vi "Collect fast fpga metadata.vi"(0 "reference in":refnum<class "metadata.lvclass">, 5 "error in (no error)":errorcluster) -> (14 "reference out":refnum<class "metadata.lvclass">, 16 "Metadata":T1, 17 "Property Names":string[](array[string]), 18 "Property values":string[](array[string]), 19 "error out":errorcluster)   [LabVIEW 2019, in "metadata.lvclass"]
uses:
  metadata.lvclass
  Metadata output --cluster.ctl
  Write time and date string --constant.ctl
panel:
  out "List property names":string
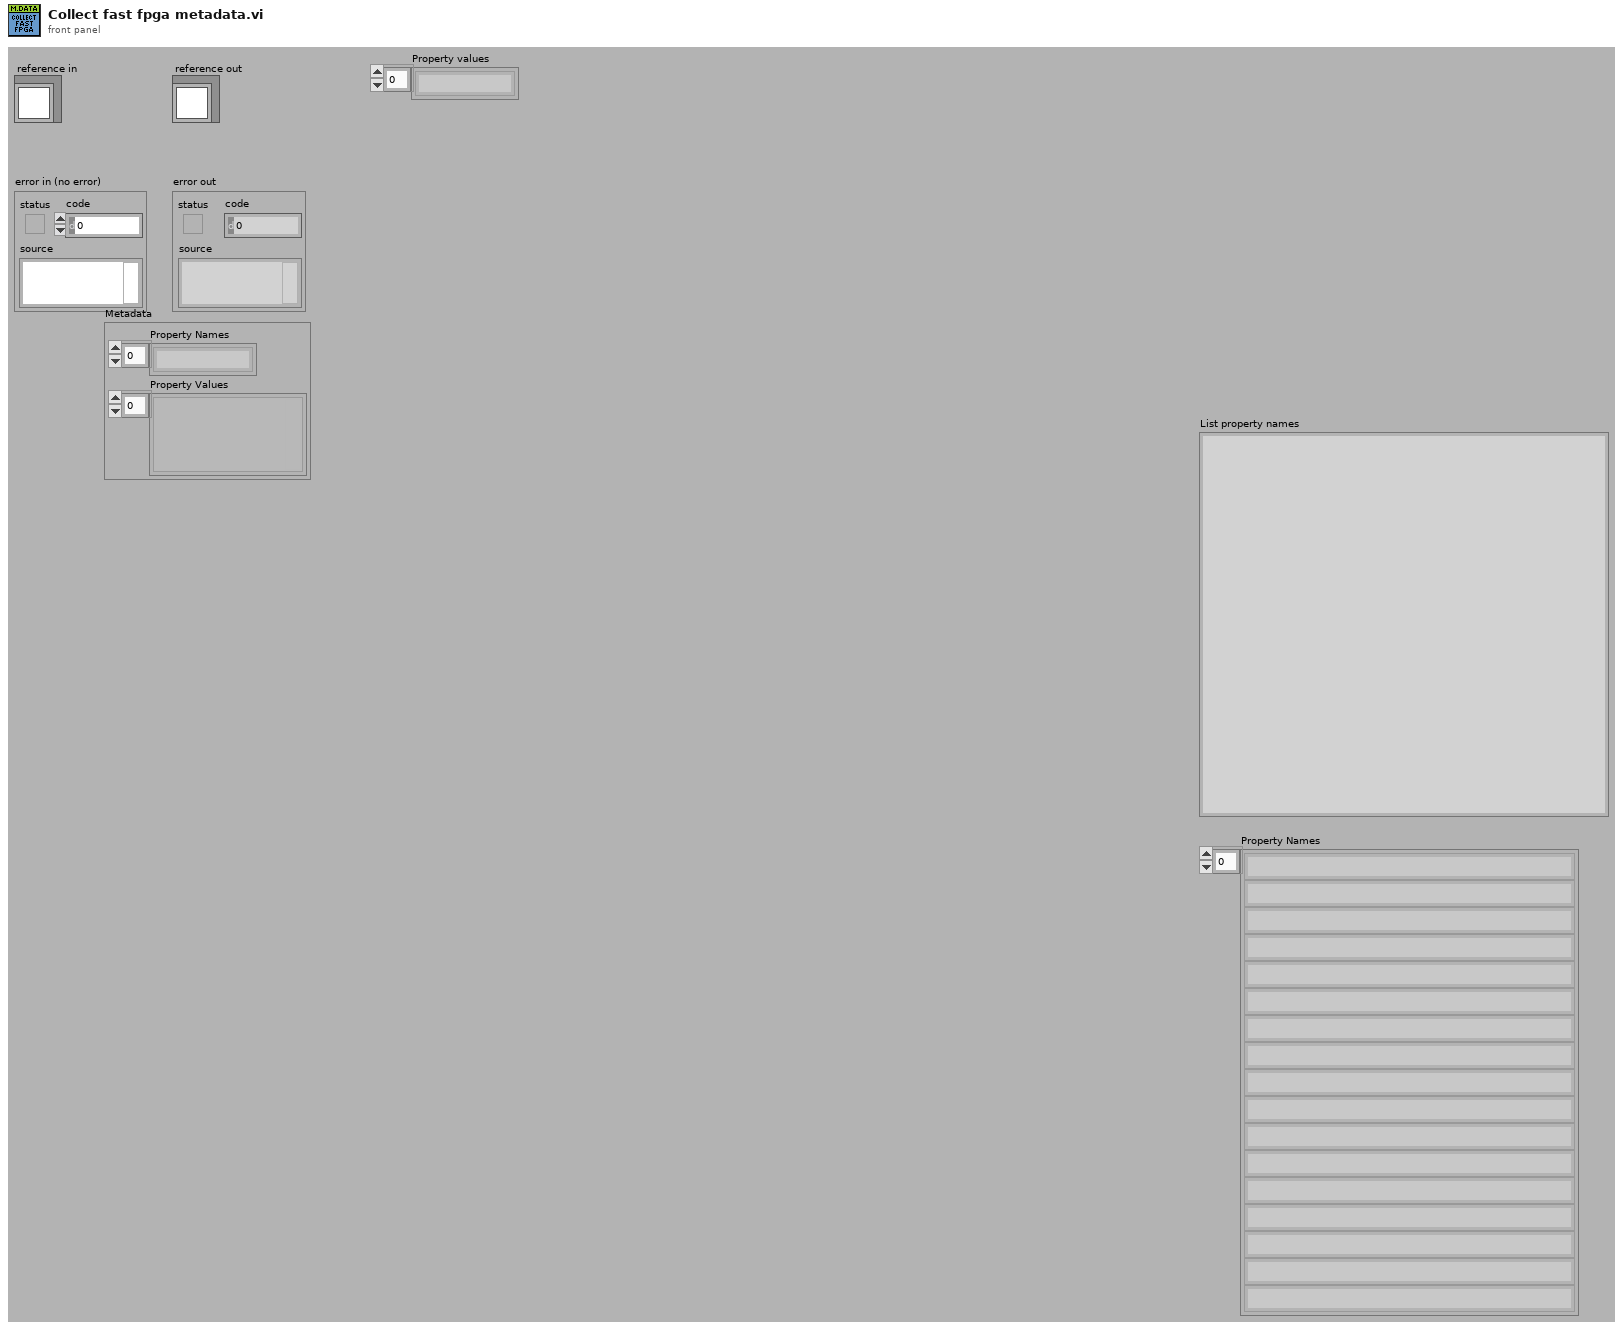
[diagram p1: front panel]
types:
  T1 = typedef "metadata.lvclass/Metadata output --cluster.ctl" = cluster{"Property Names":string[], "Property Values":variant[]}
  T2 = typedef "metadata.lvclass/Write time and date string --constant.ctl" = string
  T3 = typedef "metadata.lvclass/ObjectAttributes.ctl" = cluster{"MyAttribute":dbl, "System Control":T4, "file info":T5, "Sample info":T6, "Cantilever info":T7, "XYZ piezos":T8, "Mapping":T9, "Fcurve segment":T10[], "Fast fpga segment":T12, "Chirp":T13, "precision (6)":i16, "width (-)":i16, "Metadata":T1, "config filepath":path, "Section names []":string[], "Property names []":string[], "nb elements":u16}
  T4 = typedef "metadata.lvclass/System control parameters.ctl" = cluster{"FPGA SW version":string, "TDMS file version":string, "Instrument":string, "Instrument model":string, "Instrument scanner":string, "Instrument clockrate (Mhz)":string, "Instrument tick time (us)":string}
  T5 = typedef "metadata.lvclass/File info parameters.ctl" = cluster{"Time Stamp":timestamp, "Filename":string, "Filepath":path, "User":string, "Experiment_name":string, "Curve_id":string, "number_segments":u8, "number_consecutive_scans":u32}
  T6 = typedef "metadata.lvclass/Sample info parameters.ctl" = cluster{"Sample name":string, "Sample species":string}
  T7 = typedef "metadata.lvclass/Cantilever info parameters.ctl" = cluster{"spring constant calib method":string, "invOLS calib method":string, "thermal calib deflection channel":string, "model":string, "shape":string, "tip geometry":string, "Laser sum (V)":dbl, "Laser power (mA)":dbl, "invOLS_(nm/V)":dbl, "spring constant nominal (N/m)":dbl, "spring constant calib (N/m)":dbl, "resosnance frequency air calib (Hz)":dbl, "resosnance frequency calib (Hz)":dbl, "quality factor":dbl, "Acoefficident_GCI_(nN.s^1.3/m)":dbl, "half angle (deg)":dbl, "tip radius (m)":dbl, "tip height (m)":dbl, "system mount angle (deg)":dbl}
  T8 = typedef "metadata.lvclass/XYZ piezos parameters.ctl" = cluster{"X stage piezo sensitivity (nm/V)":dbl, "X stage piezo gain":dbl, "X velocity (V/tick)":dbl, "X closed loop":bool, "Y stage piezo sensitivity (nm/V)":dbl, "Y stage piezo gain":dbl, "Y velocity (V/tick)":dbl, "Y closed loop":bool, "Z stage piezo sensitivity (nm/V)":dbl, "Z stage piezo gain":dbl, "Z closed loop":bool, "X position (V)":dbl, "Y position (V)":dbl}
  T9 = typedef "metadata.lvclass/Mapping parameters.ctl" = cluster{"Mapping":bool, "index":u16, "position row":u16, "position column":u16, "next position row":i16, "next position column":i16, "X initial position (V)":dbl, "Y initial position (V)":dbl, "X step size (V)":dbl, "Y step size (V)":dbl}
  T10 = typedef "metadata.lvclass/Fcurve segment.ctl" = cluster{"type":T11, "fast_fpga_trigger":bool, "nb":u8, "duration (ticks)":i64, "nb points":i32, "sampling rate (S/s)":u32, "Zpiezo control out":string, "initial deflection (V)":dbl, "relative setpoint":bool, "setpoint on":bool, "setpoint (V)":dbl, "setpoint trigger channel":string, "velocity (V/tick)":dbl, "Z position setpoint trigger (V)":dbl, "Z retract length (V)":dbl, "dec factor":u32}
  T11 = typedef "metadata.lvclass/Segment type--combobox.ctl" = string
  T12 = typedef "metadata.lvclass/fast fpga segment parameters.ctl" = cluster{"Fast start time trigger":timestamp, "nb_points":u32, "sampling_rate_(S/s)":u32, "duration_(ticks)":u32}
  T13 = typedef "metadata.lvclass/Chirp added parameters.ctl" = cluster{"f start (Hz)":dbl, "f end (Hz)":dbl, "Sweep type":string}
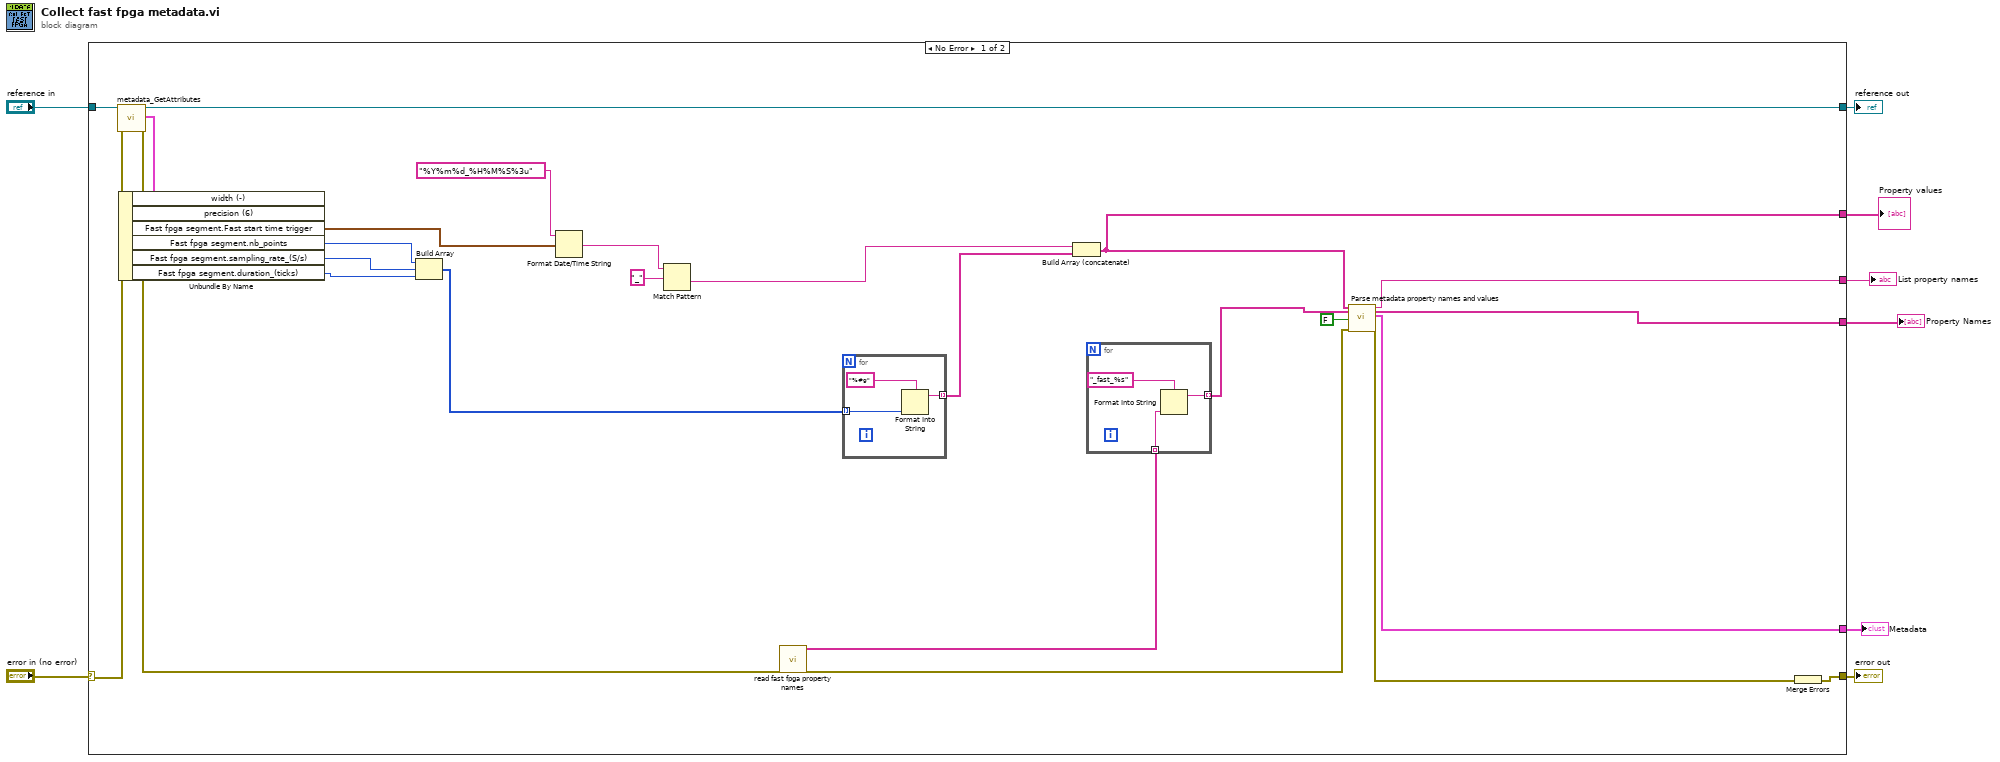
[diagram p0: block diagram]
diagram:
  n1 = case shown="No Error" "error in (no error)" {
    selector: "error in (no error)" -> [w30 w41]
    tunnel: [w33 w41] -> w7
    tunnel: [w31 w40] -> w5
    tunnel: "reference in" -> [w32 w40]
    tunnel: [w27 _] -> w4
    tunnel: [w26 _] -> w2
    tunnel: [w25 _] -> w3
    tunnel: [w11 _] -> w1
    frame No Error {
      n2 = call "metadata_GetAttributes.vi"("reference in"=w32, "error in (no error)"=w30) -> ("reference out"=w31:refnum<class "metadata.lvclass">, "attributes"=w29:T3, "error out"=w22:errorcluster)  [unwired: 14 in, 1 out]
      n3 = Unbundle By Name(w29) -> ("Fast fpga segment.Fast start time trigger"=w20:timestamp, "Fast fpga segment.nb_points"=w16:u32, "Fast fpga segment.sampling_rate_(S/s)"=w15:u32, "Fast fpga segment.duration_(ticks)"=w14:u32)  [unwired: 2 out]
      n4 = Build Array(w16, w15, w14) -> (w13:u32[])
      n5 = Format Date/Time String(time format string (%c)=T2 "%Y%m%d_%H%M%S%3u", seconds (now)=w20) -> (date/time string=w17:string)  [unwired: 1 in]
      n6 = Match Pattern(string=w17, regular expression="_") -> (after substring=w12:string)  [unwired: 1 in, 3 out]
      n7 = call "read fast fpga property names.vi"("error in (no error)"=w22) -> ("Fast fpga param"=w10:string[], "error out"=w21:errorcluster)  [unwired: 17 in]
      n8 = for {
        tunnel: [w38] -> w24 mode=indexing
        tunnel: w13 -> [w37] mode=indexing
        n9 = Format Into String(format string="%#g", w37) -> (resulting string=w38:string)  [unwired: 2 in, 1 out]
      }
      n10 = Build Array (concatenate)(w12, w24) -> (w11:string[])
      n11 = for {
        tunnel: [w35] -> w9 mode=indexing
        tunnel: w10 -> [w34] mode=indexing
        n12 = Format Into String(format string="_fast_%s", w34) -> (resulting string=w35:string)  [unwired: 2 in, 1 out]
      }
      n13 = call "Parse metadata property names and values.vi"("Data intput []"=w11, "property names []"=w9, "List param"=FALSE, "error in (no error)"=w21) -> ("Param list"=w25:string, "Array"=w27:string[], "output cluster"=w26:T1, "error out"=w28:errorcluster)  [unwired: 12 in]
      n14 = Merge Errors(w28) -> (w33:errorcluster)
    }
    frame Error {
    }
  }
  "error out" <- w7
  "reference out" <- w5
  "Property Names" <- w4
  "List property names" <- w3
  "Metadata" <- w2
  "Property values" <- w1
